vi "create_PrepLine_picture.vi"(11 "Value in":picture) -> (3 "Value out":picture)   [LabVIEW 2017]
doc: "creates the PrepLine Picture by adding the switches (according to their states) and other objects (pressure and temperature readings) to the background image"
uses:
  Classes/PrepLineObject/PrepLineObject.lvclass
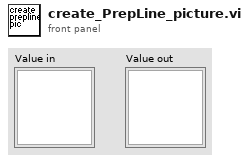
[diagram p1: front panel]
types:
  T1 = typedef "LVPoint32TypeDef.ctl" = cluster{"Horizontal":i32, "Vertical":i32}
  T2 = cluster{"Horizontal":i32, "Vertical":i32, i32, i32}
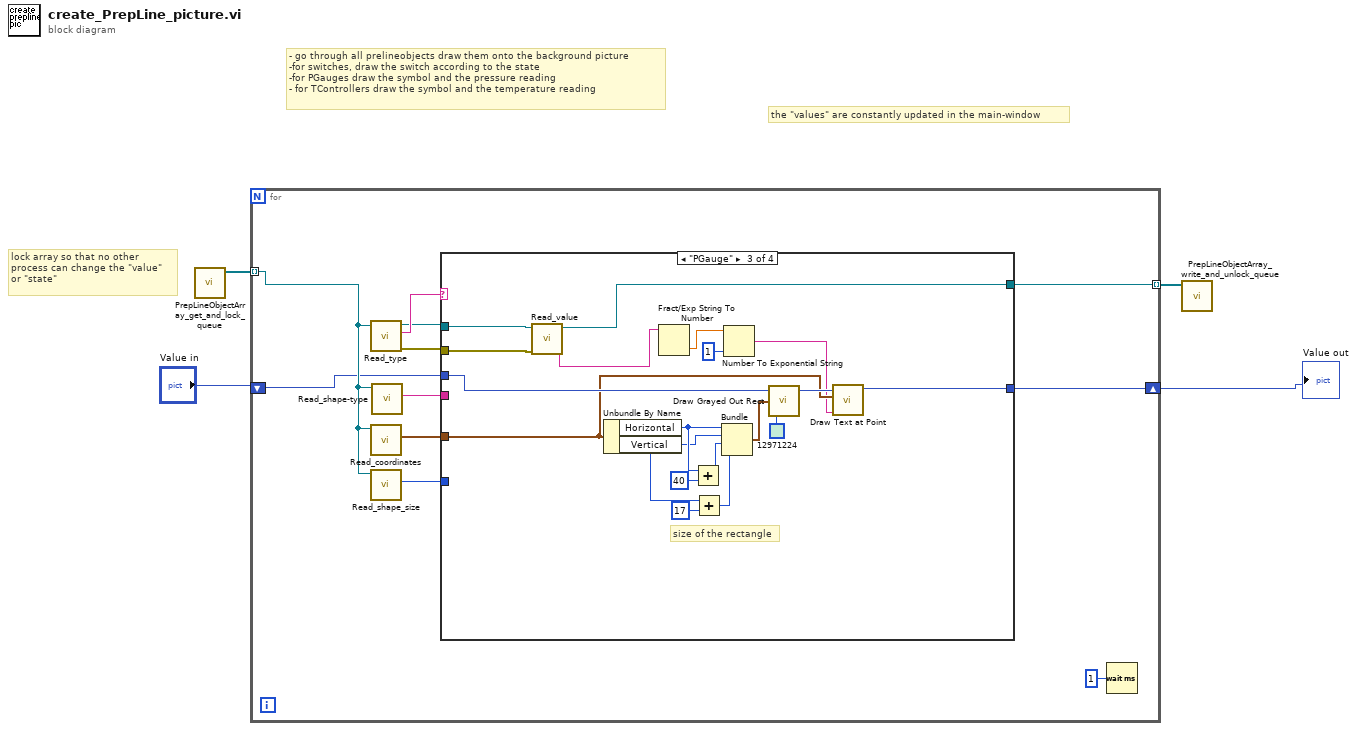
[diagram p0: block diagram]
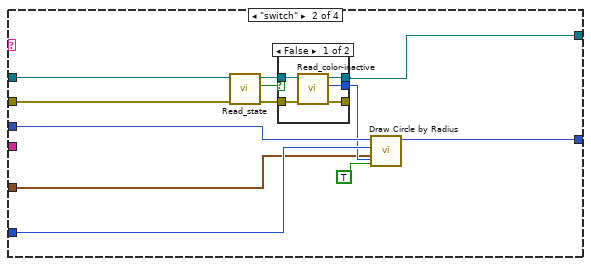
[diagram p3: hidden frame]
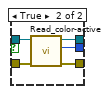
[diagram p4: hidden frame]
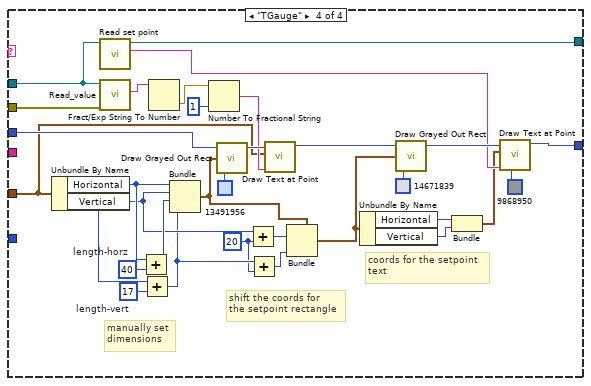
[diagram p5: hidden frame]
diagram:
  # "lock array so that no other\nprocess can change the \"value\"\nor \"state\""
  # "the \"values\" are constantly updated in the main-window"
  # "- go through all prelineobjects draw them onto the background picture\n-for switches, draw the switch according to the state\n-for PGauges draw the symbol and the pressure reading\n- for TControllers draw the symbol and the temperature reading"
  n1 = call "PrepLineObjectArray_get_and_lock_queue.vi"() -> ("PrepLineObjects"=w4:refnum<class "PrepLineObject.lvclass">[])  [unwired: 10 in, 1 out]
  n2 = for {
    shift-right: [w11] -> w1
    shift-left: "Value in" -> [w12]
    tunnel: w4 -> [w14] mode=indexing
    tunnel: [w13] -> w3 mode=indexing
    n3 = call-dynamic "Read_type.vi"("PrepLinePictureObjects in"=w14) -> ("error out"=w5:errorcluster, "type"=w8:string, "PrepLinePictureObjects out"=w6:refnum<class "PrepLineObject.lvclass">)  [unwired: 8 in]
    n4 = call-dynamic "Read_coordinates.vi"("PrepLinePictureObjects in"=w14) -> ("Coords"=w9:T1)  [unwired: 7 in, 2 out]
    n5 = call-dynamic "Read_shape_size.vi"("PrepLinePictureObjects in"=w14) -> ("shape type"=w10:i8)  [unwired: 7 in, 2 out]
    n6 = call-dynamic "Read_shape-type.vi"("PrepLineObject in"=w14) -> ("shape type"=w7:string)  [unwired: 8 in, 2 out]
    n7 = case shown="\"PGauge\"" w8 {
      tunnel: w10 -> [_ w28 _ _]
      tunnel: w12 -> [w17 w27 w58 w89]
      tunnel: [w17 w26 w50 w75] -> w11
      tunnel: w6 -> [w16 w20 w42 w59]
      tunnel: w5 -> [_ w19 w41 w61]
      tunnel: w9 -> [_ w21 w48 w72]
      tunnel: w7 -> [_ _ _ _]
      tunnel: [w16 w18 w40 w60] -> w13
      frame "False", Default {
      }
      frame "switch" {
        n8 = call-dynamic "Read_state.vi"("error in (no error)"=w19, "PrepLineObject in"=w20) -> ("error out"=w24:errorcluster, "state"=w25:bool, "PrepLineObject out"=w23:refnum<class "PrepLineObject.lvclass">)  [unwired: 7 in]
        n9 = case shown="False" w25 {
          tunnel: w24 -> [w33 w38]
          tunnel: w23 -> [w34 w39]
          tunnel: [w32 w37] -> w18
          tunnel: [w31 w36] -> _
          tunnel: [w30 w35] -> w22
          frame False {
            n10 = call-dynamic "Read_color-inactive.vi"("error in (no error)"=w33, "PrepLineObject in"=w34) -> ("error out"=w31:errorcluster, "color inactive"=w30:u32, "PrepLineObject out"=w32:refnum<class "PrepLineObject.lvclass">)  [unwired: 7 in]
          }
          frame True {
            n11 = call-dynamic "Read_color-active.vi"("error in (no error)"=w38, "PrepLineObject in"=w39) -> ("error out"=w36:errorcluster, "color active"=w35:u32, "PrepLineObject out"=w37:refnum<class "PrepLineObject.lvclass">)  [unwired: 7 in]
          }
        }
        n12 = call <vilib>:"Draw Circle by Radius.vi"("color(black)"=w22, "fill?(F)"=TRUE, "pixel center"=w21, "radius"=w28, "picture"=w27) -> ("new picture"=w26:picture)  [unwired: 6 in]
      }
      frame "PGauge" {
        # "size of the rectangle"
        n13 = call-dynamic "Read_value.vi"("error in (no error)"=w41, "PrepLineObject in"=w42) -> ("value"=w44:string, "PrepLineObject out"=w40:refnum<class "PrepLineObject.lvclass">)  [unwired: 7 in, 1 out]
        n14 = Unbundle By Name(w48) -> ("Horizontal"=w54:i32, "Vertical"=w53:i32)
        n15 = Fract/Exp String To Number(string=w44) -> (number=w46:dbl)  [unwired: 3 in, 1 out]
        n16 = Add(x=w54, y=40) -> (x+y=w52:i32)
        n17 = Add(x=w53, y=17) -> (x+y=w51:i32)
        n18 = Bundle("Horizontal"=w54, "Vertical"=w53, w52, w51) -> (w55:T2)  [unwired: 1 in]
        n19 = Number To Exponential String(number=w46, precision (6)=i16 1) -> (E-format string=w43:string)  [unwired: 2 in]
        n20 = call <vilib>:"Draw Grayed Out Rect.vi"("color(black)"=u32 12971224, "rect"=w55, "picture"=w58) -> ("new picture"=w49:picture)  [unwired: 2 in]
        n21 = call <vilib>:"Draw Text at Point.vi"("text"=w43, "origin"=w48, "picture"=w49) -> ("new picture"=w50:picture)  [unwired: 7 in, 1 out]
      }
      frame "TGauge" {
        w65 = 20 ("y")
        w87 = 17  # length-vert
        w88 = 40  # length-horz
        # "coords for the setpoint\ntext"
        # "shift the coords for\nthe setpoint rectangle"
        # "manually set\ndimensions"
        n22 = Unbundle By Name(w72) -> ("Horizontal"=w86:i32, "Vertical"=w73:i32)
        n23 = call-dynamic "Read set point.vi"("PrepLineObject in"=w59) -> ("set point"=w74:string, "PrepLineObject out"=w60:refnum<class "PrepLineObject.lvclass">)  [unwired: 8 in, 1 out]
        n24 = call-dynamic "Read_value.vi"("error in (no error)"=w61, "PrepLineObject in"=w59) -> ("value"=w82:string)  [unwired: 7 in, 2 out]
        n25 = Add(x=w86, y=w88) -> (x+y=w85:i32)
        n26 = Add(x=w73, y=w87) -> (x+y=w66:i32)
        n27 = Fract/Exp String To Number(string=w82) -> (number=w81:dbl)  [unwired: 3 in, 1 out]
        n28 = Bundle("Horizontal"=w86, "Vertical"=w73, w85, w66) -> (w68:T2)  [unwired: 1 in]
        n29 = Number To Fractional String(number=w81, precision (6)=i16 1) -> (F-format string=w79:string)  [unwired: 2 in]
        n30 = call <vilib>:"Draw Grayed Out Rect.vi"("color(black)"=u32 13491956, "rect"=w68, "picture"=w89) -> ("new picture"=w84:picture)  [unwired: 2 in]
        n31 = Add(x=w73, y=w65) -> (x+y=w67:i32)
        n32 = Add(x=w66, y=w65) -> (x+y=w64:i32)
        n33 = call <vilib>:"Draw Text at Point.vi"("text"=w79, "origin"=w72, "picture"=w84) -> ("new picture"=w76:picture)  [unwired: 7 in, 1 out]
        n34 = Bundle(cluster=w68, "Vertical"=w67, w64) -> (w63:T2)  [unwired: 2 in]
        n35 = Unbundle By Name(w63) -> ("Horizontal"=w71:i32, "Vertical"=w70:i32)
        n36 = call <vilib>:"Draw Grayed Out Rect.vi"("color(black)"=u32 14671839, "rect"=w63, "picture"=w76) -> ("new picture"=w77:picture)  [unwired: 2 in]
        n37 = Bundle("Horizontal"=w71, "Vertical"=w70) -> (w69:cluster{"Horizontal":i32, "Vertical":i32})  [unwired: 1 in]
        n38 = call <vilib>:"Draw Text at Point.vi"("text color(black)"=u32 9868950, "text"=w74, "origin"=w69, "picture"=w77) -> ("new picture"=w75:picture)  [unwired: 6 in, 1 out]
      }
    }
    n39 = Wait (ms)(milliseconds to wait=u32 1) -> ()  [unwired: 1 out]
  }
  "Value out" <- w1
  n40 = call "PrepLineObjectArray_write_and_unlock_queue.vi"("PrepLineObjArray"=w3) -> ()  [unwired: 10 in, 1 out]
